vi "SI600.vi"(0 "SI600.lvclass in":refnum<class "SI600.lvclass">, 1 "3 JEB CS951 XQ01":dbl, 2 "3 JEB CS952 XQ01":dbl, 3 "3 JEB CS953 XQ01":dbl, 4 "3 JEB CS954 XQ01":dbl, 7 "error in":errorcluster) -> (16 "RCP Speed Max":dbl, 17 "RCP Speed AVG":dbl, 18 "RCP Speed Min":dbl, 20 "SI600.lvclass out":refnum<class "SI600.lvclass">, 21 "Loop 10":T1, 22 "Loop 20":T1, 23 "Loop 30":T1, 24 "Loop 40":T1, 25 "RCP20 Speed":dbl, 27 "error out":errorcluster)   [LabVIEW 2022 SP3, in "SI600.lvclass"]
uses:
  SI600.lvclass
  SI600.lvclass/SI600.ctl
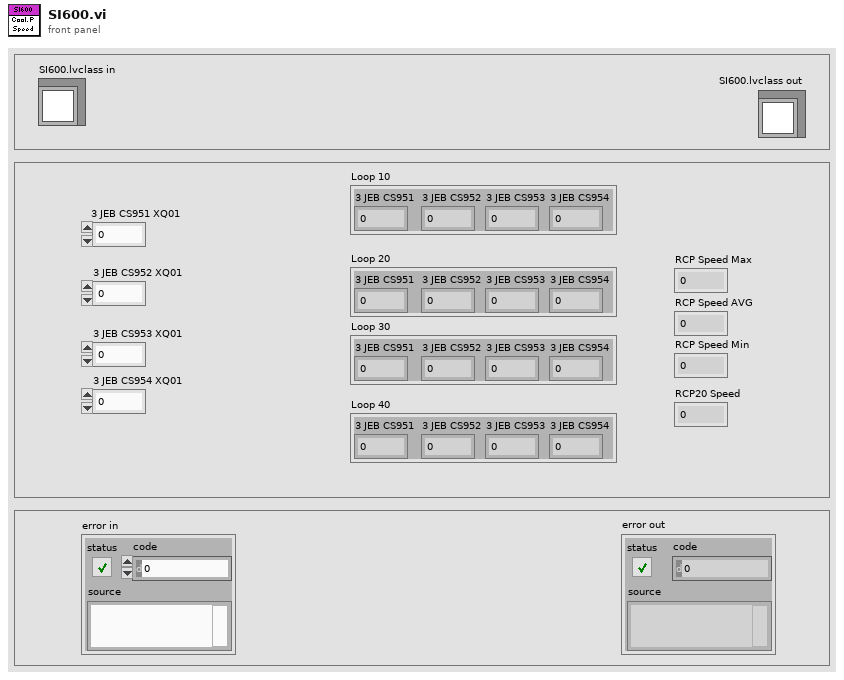
[diagram p1: front panel]
types:
  T1 = cluster{"3 JEB CS951 ":dbl, "3 JEB CS952":dbl, "3 JEB CS953":dbl, "3 JEB CS954":dbl}
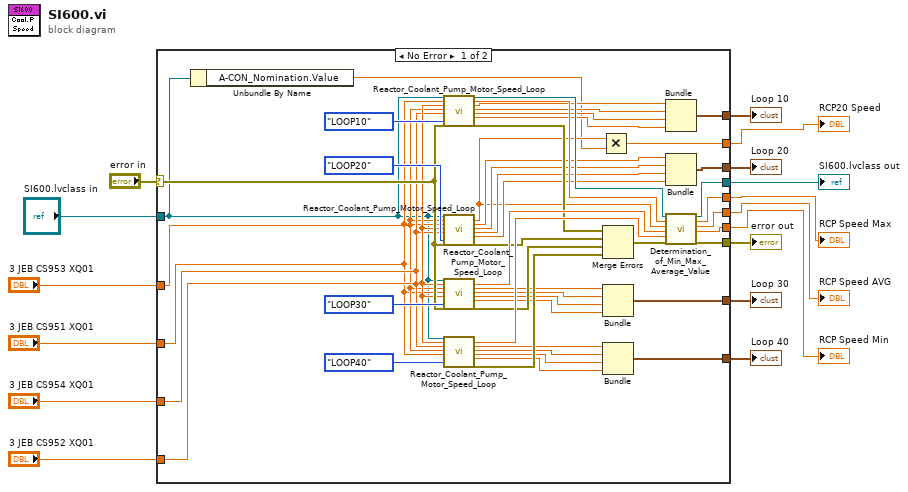
[diagram p0: block diagram]
diagram:
  n1 = case shown="No Error" "error in" {
    selector: "error in" -> [w60 w64]
    tunnel: "SI600.lvclass in" -> [w19 w65]
    tunnel: "3 JEB CS951 XQ01" -> [w55 _]
    tunnel: "3 JEB CS952 XQ01" -> [w58 _]
    tunnel: "3 JEB CS953 XQ01" -> [w56 _]
    tunnel: "3 JEB CS954 XQ01" -> [w57 _]
    tunnel: [w45 _] -> w10
    tunnel: [w44 _] -> w9
    tunnel: [w43 _] -> w8
    tunnel: [w38 _] -> w7
    tunnel: [w33 _] -> w6
    tunnel: [w28 _] -> w5
    tunnel: [w23 _] -> w4
    tunnel: [w22 w65] -> w3
    tunnel: [w21 w64] -> w2
    tunnel: [w17 _] -> w1
    frame No Error {
      n2 = Unbundle By Name(w19) -> ("A-CON_Nomination.Value"=w18:dbl)
      n3 = call "Reactor_Coolant_Pump_Motor_Speed_Loop.vi"("SI600.lvclass in"=w19, "3 JEB CS951 XQ01"=w55, "3 JEB CS952 XQ01"=w58, "3 JEB CS953 XQ01"=w56, "3 JEB CS954 XQ01"=w57, "Loop"=enum16{"LOOP10", "LOOP20", "LOOP30", "LOOP40"}."LOOP10", "error in (no error)"=w60) -> ("SI600.lvclass out"=w46:refnum<class "SI600.lvclass">, "RCP speed Loop Output"=w54:dbl, "3 JEB CS951"=w42:dbl, "3 JEB CS952"=w41:dbl, "3 JEB CS953"=w40:dbl, "3 JEB CS954"=w39:dbl, "error IO"=w51:errorcluster)  [unwired: 14 in]
      n4 = call "Reactor_Coolant_Pump_Motor_Speed_Loop.vi"("SI600.lvclass in"=w19, "3 JEB CS951 XQ01"=w56, "3 JEB CS952 XQ01"=w55, "3 JEB CS953 XQ01"=w58, "3 JEB CS954 XQ01"=w57, "Loop"=enum16{"LOOP10", "LOOP20", "LOOP30", "LOOP40"}."LOOP20", "error in (no error)"=w60) -> ("RCP speed Loop Output"=w20:dbl, "3 JEB CS951"=w37:dbl, "3 JEB CS952"=w36:dbl, "3 JEB CS953"=w35:dbl, "3 JEB CS954"=w34:dbl, "error IO"=w50:errorcluster)  [unwired: 14 in, 1 out]
      n5 = call "Reactor_Coolant_Pump_Motor_Speed_Loop.vi"("SI600.lvclass in"=w19, "3 JEB CS951 XQ01"=w57, "3 JEB CS952 XQ01"=w56, "3 JEB CS953 XQ01"=w55, "3 JEB CS954 XQ01"=w58, "Loop"=enum16{"LOOP10", "LOOP20", "LOOP30", "LOOP40"}."LOOP30", "error in (no error)"=w60) -> ("RCP speed Loop Output"=w53:dbl, "3 JEB CS951"=w32:dbl, "3 JEB CS952"=w31:dbl, "3 JEB CS953"=w30:dbl, "3 JEB CS954"=w29:dbl, "error IO"=w49:errorcluster)  [unwired: 14 in, 1 out]
      n6 = call "Reactor_Coolant_Pump_Motor_Speed_Loop.vi"("SI600.lvclass in"=w19, "3 JEB CS951 XQ01"=w58, "3 JEB CS952 XQ01"=w57, "3 JEB CS953 XQ01"=w56, "3 JEB CS954 XQ01"=w55, "Loop"=enum16{"LOOP10", "LOOP20", "LOOP30", "LOOP40"}."LOOP40") -> ("RCP speed Loop Output"=w52:dbl, "3 JEB CS951"=w27:dbl, "3 JEB CS952"=w26:dbl, "3 JEB CS953"=w25:dbl, "3 JEB CS954"=w24:dbl, "error IO"=w48:errorcluster)  [unwired: 15 in, 1 out]
      n7 = Multiply(x=w20, y=w18) -> (x*y=w17:dbl)
      n8 = Merge Errors(w51, w50, w49, w48) -> (w47:errorcluster)
      n9 = Bundle("3 JEB CS951"=w32, "3 JEB CS952"=w31, "3 JEB CS953"=w30, "3 JEB CS954"=w29) -> (w28:T1)  [unwired: 1 in]
      n10 = Bundle("3 JEB CS951"=w27, "3 JEB CS952"=w26, "3 JEB CS953"=w25, "3 JEB CS954"=w24) -> (w23:T1)  [unwired: 1 in]
      n11 = Bundle("3 JEB CS951"=w42, "3 JEB CS952"=w41, "3 JEB CS953"=w40, "3 JEB CS954"=w39) -> (w38:T1)  [unwired: 1 in]
      n12 = Bundle("3 JEB CS951"=w37, "3 JEB CS952"=w36, "3 JEB CS953"=w35, "3 JEB CS954"=w34) -> (w33:T1)  [unwired: 1 in]
      n13 = call "Determination_of_Min_Max_Average_Value.vi"("SI600.lvclass in"=w46, "RCP speed Loop 10"=w54, "RCP speed Loop 20"=w20, "RCP speed Loop 30"=w53, "RCP speed Loop 40"=w52, "error in"=w47) -> ("SI600.lvclass out"=w22:refnum<class "SI600.lvclass">, "RCP Speed Max"=w45:dbl, "RCP Speed AVG"=w44:dbl, "RCP Speed Min"=w43:dbl, "error IO"=w21:errorcluster)  [unwired: 9 in]
    }
    frame Error {
    }
  }
  "RCP Speed Max" <- w10
  "RCP Speed AVG" <- w9
  "RCP Speed Min" <- w8
  "Loop 10" <- w7
  "Loop 20" <- w6
  "Loop 30" <- w5
  "Loop 40" <- w4
  "SI600.lvclass out" <- w3
  "error out" <- w2
  "RCP20 Speed" <- w1
